vi "Write Panel Refs.vi"(8 "error in (no error)":errorcluster, 10 "Panel Refs":refnum<vi>[](array[refnum]), 11 "GUI Composition in":refnum<class "GUI Composition.lvclass">) -> (0 "error out":errorcluster, 3 "GUI Composition out":refnum<class "GUI Composition.lvclass">)   [LabVIEW 2015, in "GUI Composition.lvclass"]
uses:
  GUI Composition.lvclass
  GUI Composition.lvclass/GUI Composition.ctl
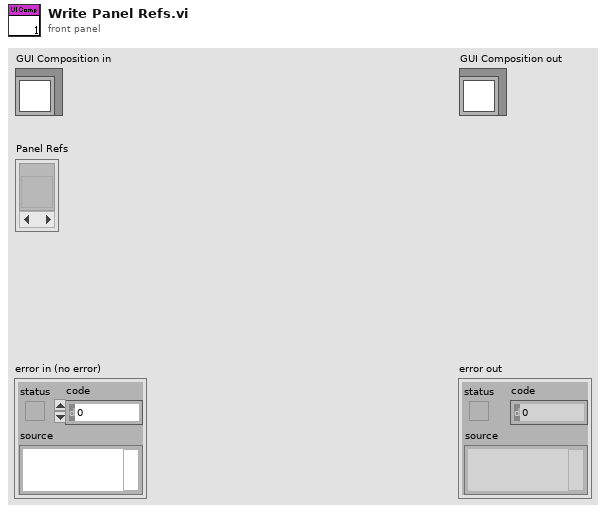
[diagram p1: front panel]
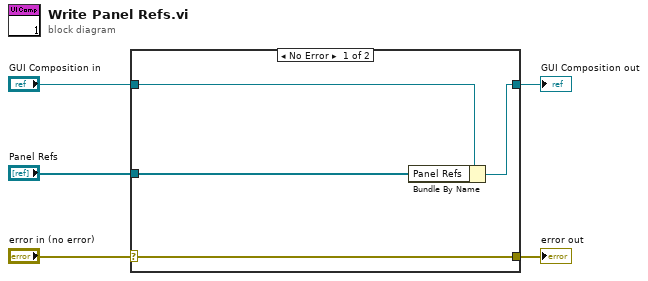
[diagram p0: block diagram]
diagram:
  n1 = case shown="No Error" "error in (no error)" {
    selector: "error in (no error)" -> [w9 w10]
    tunnel: [w9 w10] -> w4
    tunnel: [w7 w11] -> w2
    tunnel: "GUI Composition in" -> [w8 w11]
    tunnel: "Panel Refs" -> [w6 _]
    frame No Error {
      n2 = Bundle By Name(cluster=w8, "Panel Refs"=w6) -> (w7:refnum<class "GUI Composition.lvclass">)
    }
    frame Error {
    }
  }
  "error out" <- w4
  "GUI Composition out" <- w2
